vi "仿真信号的生成子程序.vi"(3 "信噪比":dbl=1.0 format="%.2p", 4 "sampling info":cluster{"Fs":dbl, "#s":dbl}={"Fs"=1000.0, "#s"=1000.0} caption="采样信息" {"Fs" format="%.2p"}, 5 "square wave \nduty cycle (%)":dbl=50.0 caption="方波占空比(%)" format="%0.2f", 6 "formula":string="sin(w*t)*sin(2*pi(1)*t)" caption="公式", 7 "相位":dbl, 8 "幅值":dbl, 9 "频率":dbl, 10 "噪声选择":enum16{"无", "均匀白噪声", "高斯噪声"}(ring), 11 "波形选择":enum16{"正弦波", "锯齿波", "三角波", "方波", "公式波"}(ring)) -> (1 "波形图":waveform(dbl)(graph))   [LabVIEW 2017]
uses:
  <vilib>/measure/NI_MABase.lvlib
  <vilib>/measure/NI_MAPro.lvlib
panel:
  # "波 形 发 生 器"
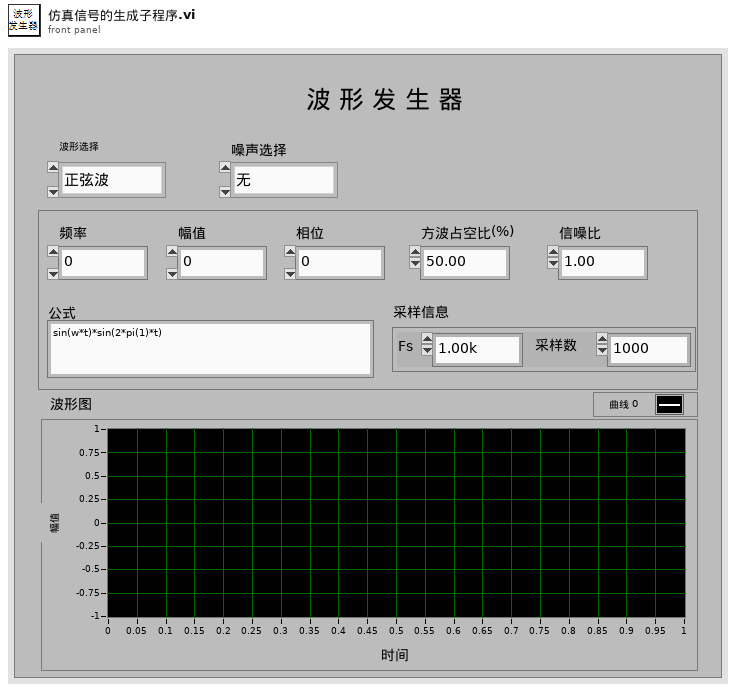
[diagram p1: front panel]
types:
  T1 = enum16{"Sine Wave", "Triangle Wave", "Square Wave", "Sawtooth Wave"}
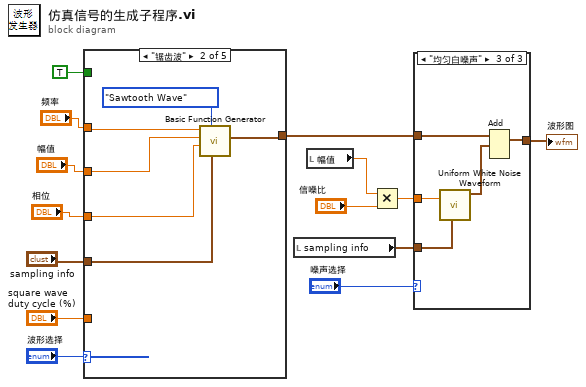
[diagram p0: block diagram]
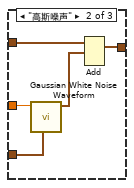
[diagram p3: hidden frame]
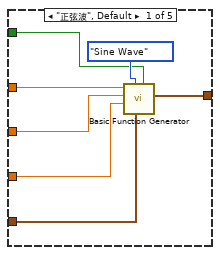
[diagram p4: hidden frame]
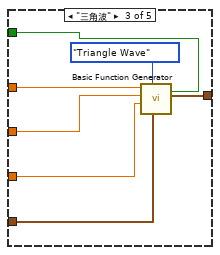
[diagram p5: hidden frame]
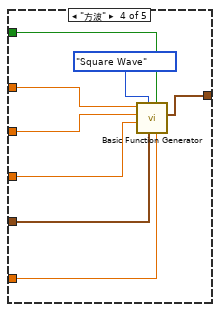
[diagram p6: hidden frame]
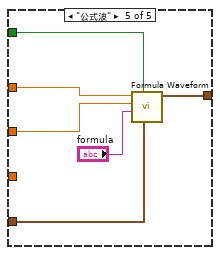
[diagram p7: hidden frame]
diagram:
  n1 = case shown="\"锯齿波\"" "波形选择" {
    tunnel: [w17 w27 w34 w36 w45] -> w12
    tunnel: "频率" -> [w20 w25 w32 w41 w48]
    tunnel: "幅值" -> [w19 w24 w31 w40 w47]
    tunnel: "相位" -> [w16 w23 w30 w39 _]
    tunnel: "sampling info" -> [w18 w22 w29 w38 w44]
    tunnel: "square wave \nduty cycle (%)" -> [_ _ _ w37 _]
    tunnel: TRUE ("reset signal") -> [w15 _ w28 w35 w43]
    frame "正弦波", Default {
      n2 = call <vilib>:"Basic Function Generator.vi"("reset signal"=w15, "sampling info"=w18, "signal type"=T1."Sine Wave", "phase"=w16, "amplitude"=w19, "frequency"=w20) -> ("signal out"=w17:waveform(dbl))  [unwired: 3 in, 2 out]
    }
    frame "锯齿波" {
      n3 = call <vilib>:"Basic Function Generator.vi"("sampling info"=w22, "signal type"=T1."Sawtooth Wave", "phase"=w23, "amplitude"=w24, "frequency"=w25) -> ("signal out"=w27:waveform(dbl))  [unwired: 4 in, 2 out]
    }
    frame "三角波" {
      n4 = call <vilib>:"Basic Function Generator.vi"("reset signal"=w28, "sampling info"=w29, "signal type"=T1."Triangle Wave", "phase"=w30, "amplitude"=w31, "frequency"=w32) -> ("signal out"=w34:waveform(dbl))  [unwired: 3 in, 2 out]
    }
    frame "方波" {
      n5 = call <vilib>:"Basic Function Generator.vi"("square wave duty cycle (%)"=w37, "reset signal"=w35, "sampling info"=w38, "signal type"=T1."Square Wave", "phase"=w39, "amplitude"=w40, "frequency"=w41) -> ("signal out"=w36:waveform(dbl))  [unwired: 2 in, 2 out]
    }
    frame "公式波" {
      n6 = call <vilib>:"Formula Waveform.vi"("sampling info"=w44, "reset signal"=w43, "formula"="formula", "amplitude"=w47, "frequency"=w48) -> ("signal out"=w45:waveform(dbl))  [unwired: 5 in, 1 out]
    }
  }
  n7 = local read "sampling info"() -> (w4:cluster{"Fs":dbl, "#s":dbl})
  n8 = local read "幅值"() -> (w13:dbl)
  n9 = Multiply(x=w13, y="信噪比") -> (x*y=w11:dbl)
  n10 = case shown="\"均匀白噪声\"" "噪声选择" {
    tunnel: [w49 w53 w56] -> w1
    tunnel: w11 -> [_ w54 w59]
    tunnel: w12 -> [w49 w52 w58]
    tunnel: w4 -> [_ w51 w55]
    frame "无", Default {
    }
    frame "高斯噪声" {
      n11 = call <vilib>:"Gaussian White Noise Waveform.vi"("sampling info"=w51, "standard deviation"=w54) -> ("signal out"=w50:waveform(dbl))  [unwired: 8 in, 1 out]
      n12 = Add(1:w50, 2:w52) -> (0:w53:waveform(dbl))  [unwired: 1 in, 1 out]
    }
    frame "均匀白噪声" {
      n13 = call <vilib>:"Uniform White Noise Waveform.vi"("sampling info"=w55, "amplitude"=w59) -> ("signal out"=w57:waveform(dbl))  [unwired: 8 in, 1 out]
      n14 = Add(1:w57, 2:w58) -> (0:w56:waveform(dbl))  [unwired: 1 in, 1 out]
    }
  }
  "波形图" <- w1
